vi "FetchServoTraceResults.vi"(8 "error in":errorcluster, 9 "NumberAveragesCaptured":i32=100, 10 "rfsgSession":refnum<k15>, 11 "ServoSessionIn":u32) -> (0 "error out":errorcluster, 2 "Servo Results":T1={"Final Input Power (dBm)"=0.05, "Final Output Power (dBm)"=0.05, "Calculated Dut Gain (dB)"=0.05, "Servo Trace"=[]}, 3 "ServoSessionOut":u32)   [LabVIEW 2016, in "Power Servo.lvlib"]
uses:
  Power Servo.lvlib
  Type Definitions/ServoResult.ctl
  Type Definitions/Enable.ctl
  <userlib>/_NI Power Servoing IP/HostRdl/NI Power Servoing IP New (Host).lvlib
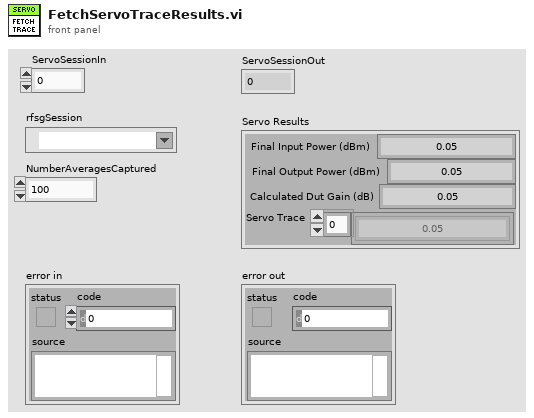
[diagram p1: front panel]
types:
  T1 = typedef "Power Servo.lvlib/ServoResult.ctl" = cluster{"Final Input Power (dBm)":dbl, "Final Output Power (dBm)":dbl, "Calculated Dut Gain (dB)":dbl, "Servo Trace":dbl[]}
  T2 = typedef "Power Servo.lvlib/Enable.ctl" = enum16{"False", "True"}
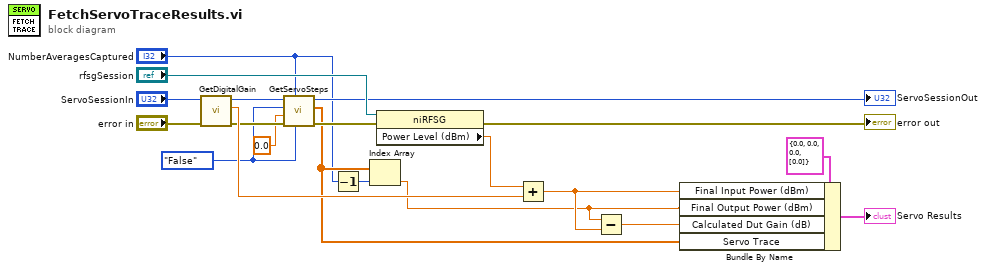
[diagram p0: block diagram]
diagram:
  w6 = Enable."False" ("Enable")
  n1 = call <userlib>:"GetDigitalGain.vi"("error in"="error in", "SessionHandleIn"="ServoSessionIn") -> ("error out"=w8:errorcluster, "DigitalGainDB"=w15:dbl, "SessionHandleOut"=w10:u32)  [unwired: 6 in, 1 out]
  n2 = call <userlib>:"GetServoSteps.vi"("CaptureAfterLeveling"=w6, "NumberAveragesCaptured"="NumberAveragesCaptured", "error in"=w8, "ExtraTimeS"=0.0, "Continuous"=w6, "SessionHandleIn"=w10) -> ("error out"=w7:errorcluster, "MeasurementLevels"=w4:dbl[], "SessionHandleOut"=→"ServoSessionOut":u32)  [unwired: 2 in, 1 out]
  n3 = Decrement(x="NumberAveragesCaptured") -> (x-1=w3:i32)
  n4 = Index Array(array=w4, index=w3) -> (element=w1:dbl)
  n5 = property class="niRFSG"(reference="rfsgSession", error in=w7) -> (error out=→"error out":errorcluster, "Power Level (dBm)"=w16:dbl)  [unwired: 1 out]
  n6 = Add(x=w16, y=w15) -> (x+y=w13:dbl)
  n7 = Subtract(x=w1, y=w13) -> (x-y=w12:dbl)
  n8 = Bundle By Name(cluster=T1 {"Final Input Power (dBm)"=0.0, "Final Output Power (dBm)"=0.0, "Calculated Dut Gain (dB)"=0.0, "Servo Trace"=[0.0]} ("Servo Result"), "Final Input Power (dBm)"=w13, "Final Output Power (dBm)"=w1, "Calculated Dut Gain (dB)"=w12, "Servo Trace"=w4) -> (→"Servo Results":T1)
